vi "Clamp Vertical Min VI.vi"(0 "Image":T3, 2 "Rectangle":T5 {"Rotation" format="%.2f"; "Left" scale=0.0..1024.0; "Right" scale=0.0..1024.0}, 3 "Coordinate System":T4 {"Measurement System"."Axis Reference" items=["Direct", "Indirect"]; "Measurement System"."Angle (deg)" format="%.2f"; "Measurement System"."Origin"."Y" format="%.2f"; "Measurement System"."Origin"."X" format="%.2f"; "Reference System"."Axis Reference" items=["Direct", "Indirect"]; "Reference System"."Angle (deg)" format="%.2f"; "Reference System"."Origin"."Y" format="%.2f"; "Reference System"."Origin"."X" format="%.2f"}, 5 "error in (no error)":errorcluster, 8 "Settings":T2={"Contrast"=40, "Filter width"=4, "Steepness"=2, "Subsampling Ratio"=5, "Show Search Area"=FALSE, "Show Search Lines"=FALSE, "Show Edges Found"=FALSE, "Show Result"=TRUE}) -> (7 "Line Coordinates":T1(array[cluster]) {"?"."Y" format="%.2f"; "?"."X" format="%.2f"; "?"."Y" format="%.2f"; "?"."X" format="%.2f"}, 9 "appended array":cluster{"X":sgl, "Y":sgl}[](array[cluster]), 10 "Edge Coordinates":cluster{"X":sgl, "Y":sgl}[](array[cluster]) {"Y" format="%.2f"; "X" format="%.2f"}, 11 "Perpendicular Lines":T1(array[cluster])=[{{"X"=55.0, "Y"=48.0}, {"X"=263.0, "Y"=104.0}}, {{"X"=53.0, "Y"=53.0}, {"X"=262.0, "Y"=109.0}}, {{"X"=52.0, "Y"=58.0}, {"X"=261.0, "Y"=113.0}}, {{"X"=51.0, "Y"=62.0}, {"X"=259.0, "Y"=118.0}}, {{"X"=49.0, "Y"=67.0}, {"X"=258.0, "Y"=123.0}}, {{"X"=48.0, "Y"=72.0}, {"X"=257.0, "Y"=128.0}}, {{"X"=47.0, "Y"=77.0}, {"X"=255.0, "Y"=133.0}}, {{"X"=46.0, "Y"=82.0}, {"X"=254.0, "Y"=138.0}}, {{"X"=44.0, "Y"=87.0}, {"X"=253.0, "Y"=142.0}}, {{"X"=43.0, "Y"=91.0}, {"X"=252.0, "Y"=147.0}}, {{"X"=42.0, "Y"=96.0}, {"X"=250.0, "Y"=152.0}}] {"?"."Y" format="%.2f"; "?"."X" format="%.2f"; "?"."Y" format="%.2f"; "?"."X" format="%.2f"}, 13 "Points":cluster{"X":sgl, "Y":sgl}[](array[cluster])=[{"X"=67.0, "Y"=51.0}, {"X"=230.0, "Y"=95.0}, {"X"=66.0, "Y"=56.0}, {"X"=230.0, "Y"=100.0}, {"X"=66.0, "Y"=62.0}, {"X"=230.0, "Y"=105.0}, {"X"=66.0, "Y"=66.0}, {"X"=230.0, "Y"=110.0}, {"X"=65.0, "Y"=71.0}, {"X"=230.0, "Y"=115.0}, {"X"=65.0, "Y"=77.0}, {"X"=230.0, "Y"=121.0}, {"X"=65.0, "Y"=82.0}, {"X"=229.0, "Y"=126.0}, {"X"=65.0, "Y"=87.0}, {"X"=229.0, "Y"=131.0}, {"X"=64.0, "Y"=92.0}, {"X"=229.0, "Y"=136.0}, {"X"=64.0, "Y"=97.0}, {"X"=229.0, "Y"=141.0}, {"X"=64.0, "Y"=102.0}, {"X"=229.0, "Y"=146.0}] {"Y" format="%.2f"; "X" format="%.2f"}, 14 "Image Out":T3, 16 "Distance":sgl format="%.2f", 17 "Coordinate System (duplicate)":T4 {"Measurement System"."Axis Reference" items=["Direct", "Indirect"]; "Measurement System"."Angle (deg)" format="%.2f"; "Measurement System"."Origin"."Y" format="%.2f"; "Measurement System"."Origin"."X" format="%.2f"; "Reference System"."Axis Reference" items=["Direct", "Indirect"]; "Reference System"."Angle (deg)" format="%.2f"; "Reference System"."Origin"."Y" format="%.2f"; "Reference System"."Origin"."X" format="%.2f"}, 19 "error out":errorcluster)   [LabVIEW 2019]
uses:
  <vilib>/vision/Image Controls.llb/IMAQ Image.ctl
  <vilib>/vision/NI_Vision_Development_Module.lvlib
panel:
  out "Elapsed time (ms)":u32
  # "Start Point"
  # "End Point"
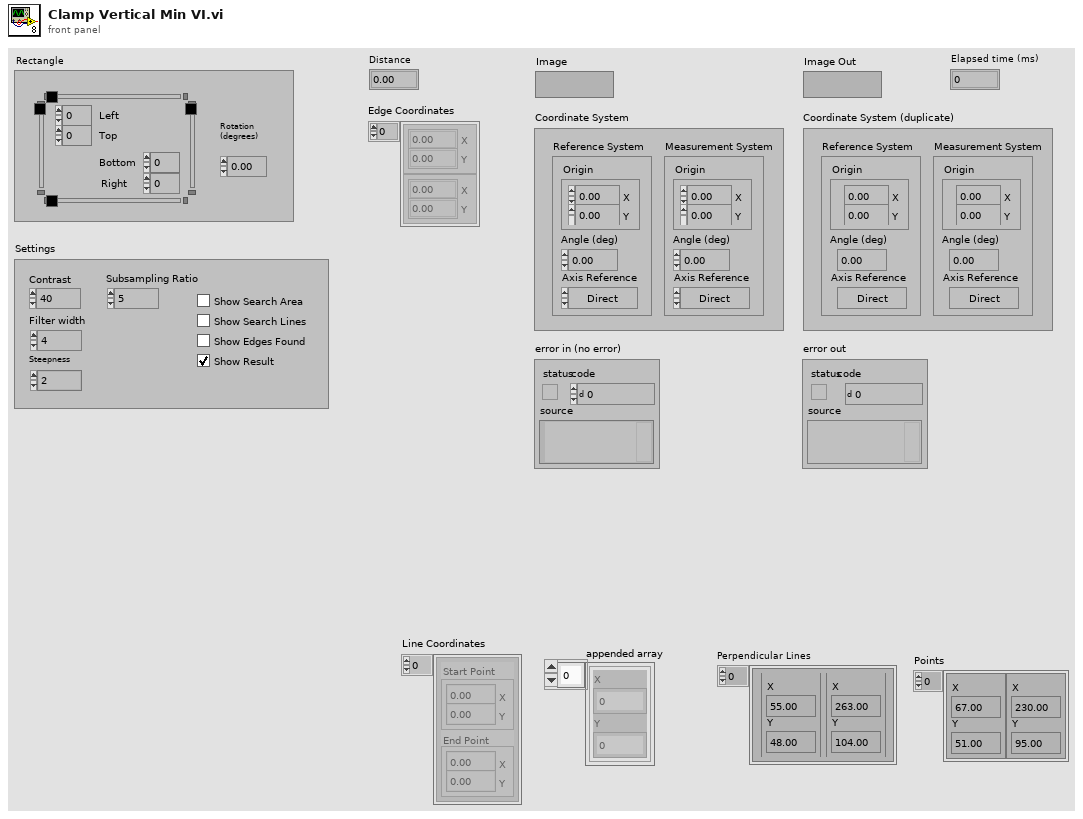
[diagram p1: front panel]
types:
  T1 = cluster{cluster{"X":sgl, "Y":sgl}, cluster{"X":sgl, "Y":sgl}}[]
  T2 = cluster{"Contrast":i32, "Filter width":i32, "Steepness":i32, "Subsampling Ratio":u32, "Show Search Area":bool, "Show Search Lines":bool, "Show Edges Found":bool, "Show Result":bool}
  T3 = typedef "IMAQ Image.ctl" = refnum<image>
  T4 = typedef "IMAQ Coordinate System" = cluster{"Reference System":cluster{"Origin":cluster{"X":sgl, "Y":sgl}, "Angle (deg)":sgl, "Axis Reference":u32}, "Measurement System":cluster{"Origin":cluster{"X":sgl, "Y":sgl}, "Angle (deg)":sgl, "Axis Reference":u32}}
  T5 = typedef "IMAQ Rectangle" = cluster{"Left":i32, "Top":i32, "Right":i32, "Bottom":i32, "Rotation":dbl}
  T6 = cluster{"Origin":cluster{"X":sgl, "Y":sgl}, "Angle (deg)":sgl, "Axis Reference":u32}
  T7 = typedef "ROI Descriptor" = cluster{"Global Rectangle":i32[], "Contours":cluster{"ID":enum32{"External", "Internal"}, "Type":u32, "Coordinates":i32[]}[]}
  T8 = cluster{"Global Rectangle":i32[], "Contours":cluster{"ID":enum32{"External", "Internal"}, "Type":u32, "Coordinates":i32[]}[]}
  T9 = cluster{"Interpolation Type":enum32{"", "Quadratic", "Cubic Spline"}, "SubPixel Accuracy":enum32{"None", "One Half", "One Third", "One Fourth", "One Fifth", "One Sixth", "One Seventh", "One Eight", "One Ninth", "One Tenth", "One Eleventh", "One Twelveth"}}
  T10 = enum32{"Get First Edge", "Get First + Last Edge", "Get All Edges"}
  T11 = cluster{"Contrast":i32, "Filter width":i32, "Steepness":i32}
  T12 = cluster{cluster{"X":sgl, "Y":sgl}, cluster{"X":sgl, "Y":sgl}}
  T13 = cluster{"Show Search Area":bool, "Show Search Lines":bool, "Show Edges Found":bool, "Show Result":bool}
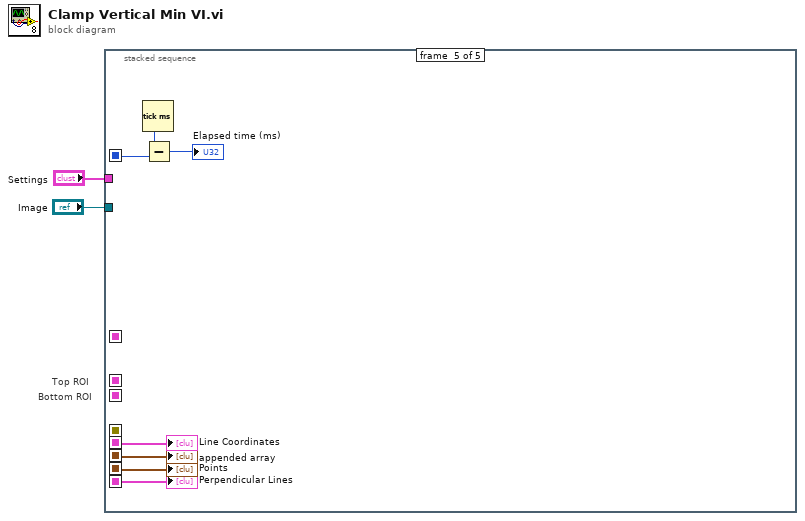
[diagram p0: block diagram]
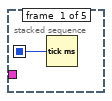
[diagram p2: hidden frame]
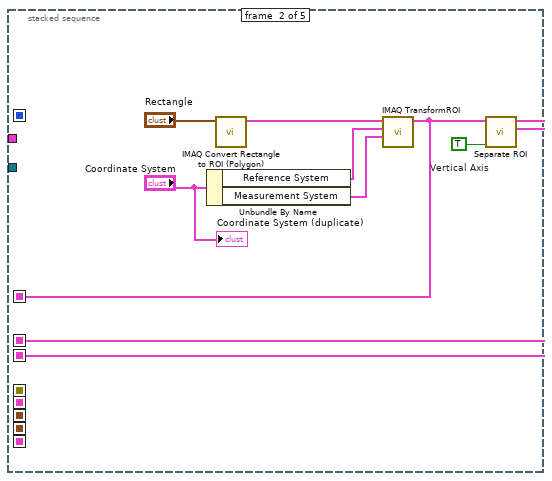
[diagram p3: hidden frame]
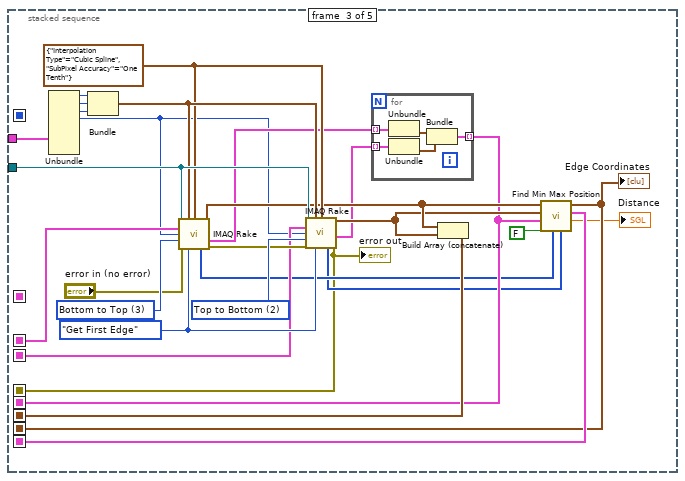
[diagram p4: hidden frame]
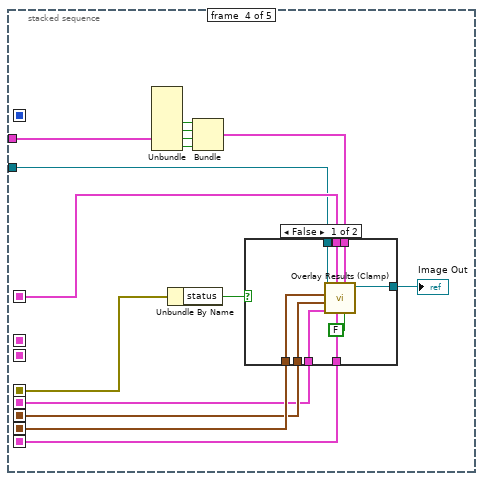
[diagram p5: hidden frame]
diagram:
  # "Bottom ROI"
  # "Top ROI"
  n1 = stacked-sequence {
    seq-local: [_ _ w33 _ _] -> [_ _ _ w60 w72]
    seq-local: [w3 _ _ _ _] -> [_ _ _ _ w77]
    seq-local: [_ _ w34 _ _] -> [_ _ _ w59 w73]
    seq-local: [_ _ w16 _ _] -> [_ _ _ w58 w74]
    seq-local: [_ _ w35 _ _] -> [_ _ _ w52 w71]
    seq-local: [_ w10 _ _ _] -> [_ _ w23 _ _]
    seq-local: [_ w9 _ _ _] -> [_ _ w22 _ _]
    seq-local: [_ w7 _ _ _] -> [_ _ _ w50 _]
    seq-local: [_ _ w13 _ _] -> [_ _ _ w47 _]
    tunnel: "Image" -> [_ _ w28 w49 _]
    tunnel: "Settings" -> [_ _ w36 w53 _]
    frame #0 {
      n2 = Tick Count (ms)() -> (millisecond timer value=w3:u32)
    }
    frame #1 {
      w8 = TRUE  # Vertical Axis
      # "Find Edges"
      n3 = Unbundle By Name("Coordinate System") -> ("Reference System"=w5:T6, "Measurement System"=w4:T6)
      n4 = call "IMAQ Convert Rectangle to ROI (Polygon)"("Rectangle"="Rectangle") -> ("ROI Descriptor"=w12:T7)  [unwired: 1 in, 8 out]
      n5 = call "IMAQ TransformROI"("New Reference"=w4, "Base Reference"=w5, "ROI Descriptor"=w12) -> ("ROI Descriptor out"=w7:T7)  [unwired: 1 in, 7 out]
      n6 = call <vilib>:"Separate ROI.vi"("Axis"=w8, "ROI Descriptor"=w7) -> ("Right/Bottom ROI"=w9:T8, "Left/Top ROI"=w10:T8)  [unwired: 4 out]
      "Coordinate System (duplicate)" <- "Coordinate System"
    }
    frame #2 {
      w29 = u32 2 items=["Left to Right", "Right to Left", "Top to Bottom", "Bottom to Top"]
      w26 = T9 {"Interpolation Type"=enum."Cubic Spline", "SubPixel Accuracy"=enum."One Tenth"} ("SubPixel Information")
      w31 = T10."Get First Edge" ("Process")
      w30 = u32 3 items=["Left to Right", "Right to Left", "Top to Bottom", "Bottom to Top"]
      # "Find Edges"
      n7 = Unbundle(w36) -> ("Contrast"=w38:i32, "Filter width"=w39:i32, "Steepness"=w40:i32, "Subsampling Ratio"=w18:u32)  [unwired: 4 out]
      n8 = Bundle("Contrast"=w38, "Filter width"=w39, "Steepness"=w40) -> (w27:T11)  [unwired: 1 out]
      n9 = call "IMAQ Rake"("Image"=w28, "Edge Parameters"=w27, "SubPixel Information"=w26, "ROI Descriptor"=w23, "Step Size"=w18, "Scan Direction"=w30, "error in (no error)"="error in (no error)", "Process"=w31) -> ("First Edges"=w21:cluster{"X":sgl, "Y":sgl}[], "Line Coordinates"=w19:T1, "Lines with Edges"=w15:u32[], "error out"=w24:errorcluster)  [unwired: 1 in, 3 out]
      n10 = call "IMAQ Rake"("Image"=w28, "Edge Parameters"=w27, "SubPixel Information"=w26, "ROI Descriptor"=w22, "Step Size"=w18, "Scan Direction"=w29, "error in (no error)"=w24, "Process"=w31) -> ("First Edges"=w20:cluster{"X":sgl, "Y":sgl}[], "Line Coordinates"=w17:T1, "Lines with Edges"=w14:u32[], "error out"=w13:errorcluster)  [unwired: 1 in, 3 out]
      "error out" <- w13
      n11 = for {
        tunnel: w19 -> [w45] mode=indexing
        tunnel: w17 -> [w44] mode=indexing
        tunnel: [w41] -> w16 mode=indexing
        n12 = Unbundle(w45) -> (w43:cluster{"X":sgl, "Y":sgl})  [unwired: 1 out]
        n13 = Unbundle(w44) -> (w42:cluster{"X":sgl, "Y":sgl})  [unwired: 1 out]
        n14 = Bundle(w43, w42) -> (w41:T12)  [unwired: 1 out]
      }
      n15 = Build Array (concatenate)(w21, w20) -> (w34:cluster{"X":sgl, "Y":sgl}[])
      n16 = call <vilib>:"Find Min Max Position.vi"("Lines with Edges (last)"=w14, "Lines with Edges (first)"=w15, "Min / Max"=FALSE, "Search Lines"=w16, "Last Edges"=w20, "First Edges"=w21) -> ("Distance"=→"Distance":sgl, "Perpendicular Lines"=w35:T1, "Points"=w33:cluster{"X":sgl, "Y":sgl}[])  [unwired: 3 out]
      "Edge Coordinates" <- w33
    }
    frame #3 {
      # "Update Overlay"
      n17 = Unbundle(w53) -> ("Show Search Area"=w57:bool, "Show Search Lines"=w56:bool, "Show Edges Found"=w55:bool, "Show Result"=w54:bool)  [unwired: 4 out]
      n18 = Unbundle By Name(w47) -> ("status"=w46:bool)
      n19 = Bundle("Show Search Area"=w57, "Show Search Lines"=w56, "Show Edges Found"=w55, "Show Result"=w54) -> (w51:T13)  [unwired: 1 out]
      n20 = case shown="False" w46 {
        tunnel: w60 -> [w69 _]
        tunnel: w59 -> [w68 _]
        tunnel: w58 -> [w67 _]
        tunnel: w52 -> [w66 _]
        tunnel: w51 -> [w64 _]
        tunnel: w50 -> [w63 _]
        tunnel: w49 -> [w62 w70]
        tunnel: [w61 w70] -> w48
        frame False {
          n21 = call <vilib>:"Overlay Results (Clamp).vi"("Min / Max"=FALSE, "Setup"=w64, "Perpendicular Lines"=w66, "ROI Descriptor"=w63, "Search Lines"=w67, "All Edges Found"=w68, "Measurement Edges"=w69, "Image In"=w62) -> ("Image Out"=w61:T3)  [unwired: 3 out]
        }
        frame True {
        }
      }
      "Image Out" <- w48
    }
    frame #4 {
      n22 = Tick Count (ms)() -> (millisecond timer value=w76:u32)
      n23 = Subtract(x=w76, y=w77) -> (x-y=→"Elapsed time (ms)":u32)
      "Line Coordinates" <- w74
      "appended array" <- w73
      "Points" <- w72
      "Perpendicular Lines" <- w71
    }
  }
